vi "Sub_Connect_FGV.vi"(6 "timeout ms (20000)":i32=20000, 7 "MQTT Broker":cluster{"address (IP)":string, "port":u16}={"address (IP)"="broker.mqttdashboard.com", "port"=1883}, 8 "error in":errorcluster, 10 "Command":T1) -> (0 "error out":errorcluster, 3 "MQTT ref out":refnum<k5>)   [LabVIEW 2019, in "MQTT_Functions.lvlib"]
uses:
  MQTT_Functions.lvlib
  Controls/Conn_FGV_Cmds.ctl
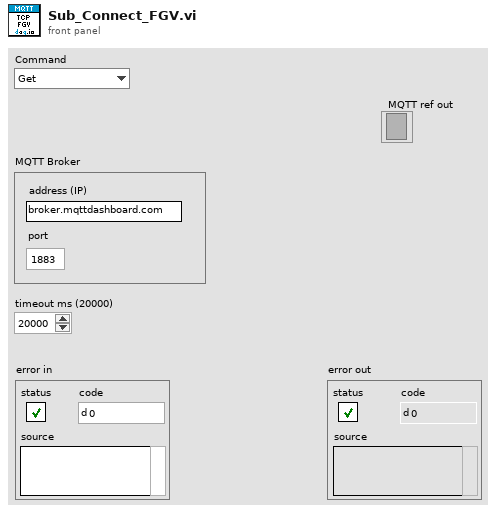
[diagram p1: front panel]
types:
  T1 = typedef "MQTT_Functions.lvlib/Conn_FGV_Cmds.ctl" = enum16{"Get", "Set", "Delete"}
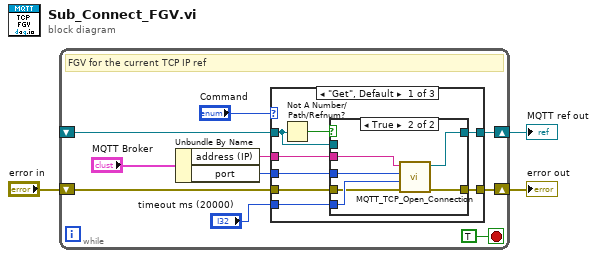
[diagram p0: block diagram]
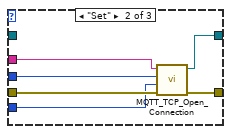
[diagram p3: hidden frame]
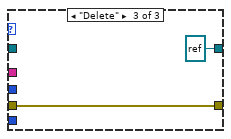
[diagram p4: hidden frame]
diagram:
  n1 = while {
    shift-right: [w7] -> w1
    shift-left: "error in" -> [w8]
    shift-right: [w6] -> w3
    shift-left: _ -> [w5]
    stop <- TRUE stop-if-true
    # "FGV for the current TCP IP ref"
    n2 = Unbundle By Name("MQTT Broker") -> ("address (IP)"=w10:string, "port"=w9:u16)
    n3 = case shown="\"Get\", Default" "Command" {
      tunnel: w10 -> [w20 w35 _]
      tunnel: w9 -> [w19 w34 _]
      tunnel: w8 -> [w17 w33 w36]
      tunnel: [w16 w32 w36] -> w7
      tunnel: [w15 w31 refnum<k5> refnum ("connection ID")] -> w6
      tunnel: w5 -> [w14 _ _]
      tunnel: "timeout ms (20000)" -> [w18 w30 _]
      frame "Get", Default {
        n4 = Not A Number/Path/Refnum?(number/path/refnum=w14) -> (NaN/Path/Refnum?=w21:bool)
        n5 = case shown="True" w21 {
          tunnel: w20 -> [_ w29]
          tunnel: w19 -> [_ w28]
          tunnel: w18 -> [_ w27]
          tunnel: w17 -> [w22 w26]
          tunnel: [w22 w25] -> w16
          tunnel: [w23 w24] -> w15
          tunnel: w14 -> [w23 _]
          frame False {
            # "existing refnum\nis likely good"
          }
          frame True {
            n6 = call "MQTT_TCP_Open_Connection.vi"("error in (no error)"=w26, "timeout ms (20000)"=w27, "remote port or service name"=w28, "address"=w29) -> ("error out"=w25:errorcluster, "connection ID"=w24:refnum<k5>)  [unwired: 6 in]
          }
        }
      }
      frame "Set" {
        n7 = call "MQTT_TCP_Open_Connection.vi"("error in (no error)"=w33, "timeout ms (20000)"=w30, "remote port or service name"=w34, "address"=w35) -> ("error out"=w32:errorcluster, "connection ID"=w31:refnum<k5>)  [unwired: 6 in]
      }
      frame "Delete" {
      }
    }
  }
  "MQTT ref out" <- w3
  "error out" <- w1
